vi "02 - Basic and Advanced DSP.vi"   [LabVIEW 2021]
uses:
  <vilib>/Analysis/NI_AALBase.lvlib
  <vilib>/Analysis/NI_AALPro.lvlib
  <vilib>/Analysis/NI_AAL_SigProc.lvlib
  <vilib>/gmath/NI_Gmath.lvlib
  <vilib>/addons/Digital Filter Design/NI_DigFilterLicensed.lvlib
  <vilib>/addons/_Advanced Signal Processing/NI_AdvSigProcTFA.lvlib
  <vilib>/addons/_Advanced Signal Processing/NI_AdvSigProcWA.lvlib
  <vilib>/addons/_Advanced Signal Processing/NI_AdvSigProcTSA.lvlib
  <vilib>/addons/Time Series Analysis/Correlation and Spectral Analysis.llb/TSA MUSIC (Waveform).vi
  <vilib>/Analysis/2dsp.llb/1D Convolution (DBL).vi
  <vilib>/Analysis/4window.llb/Hanning Window (DBL).vi
  <vilib>/Analysis/2dsp.llb/1D Cross Correlation (DBL).vi
  <vilib>/Analysis/3filter.llb/Chebyshev Filter (DBL).vi
  <vilib>/Analysis/2dsp.llb/Power Spectrum (DBL).vi
  <vilib>/Analysis/4window.llb/Blackman-Harris Window (DBL).vi
  <vilib>/addons/Wavelet Analysis/continuous wavelet transform.llb/WA Continuous Wavelet Transform (Waveform).vi
  <vilib>/addons/Time Frequency Analysis/Spectrogram.llb/TFA Online STFT Spectrogram (Waveform).vi
  <vilib>/addons/Time Frequency Analysis/Spectrogram.llb/TFA Choi-Williams Distribution (Waveform).vi
  <vilib>/addons/Time Series Analysis/Correlation and Spectral Analysis.llb/TSA Bispectrum (Waveform).vi
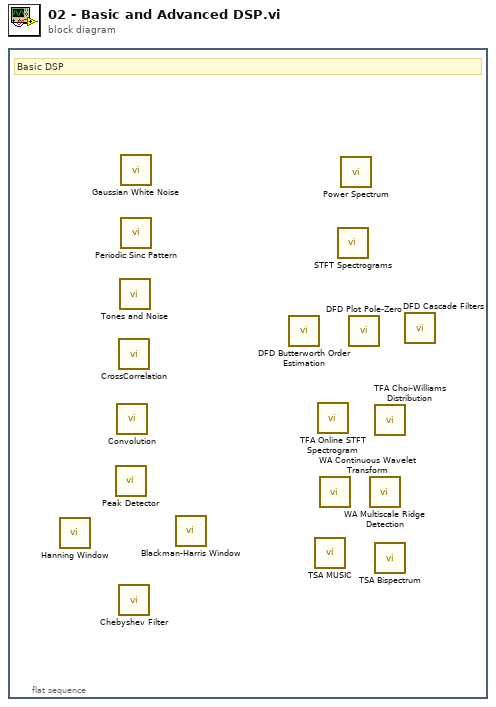
[diagram p0: block diagram]
diagram:
  n1 = flat-sequence {
    frame #0 {
      # "Basic DSP"
      n2 = call-poly <vilib>:"Hanning Window.vi"() -> ()  [unwired: 1 in, 2 out]
      n3 = call <vilib>:"Peak Detector.vi"() -> ()  [unwired: 7 in, 5 out]
      n4 = call-poly <vilib>:"Convolution.vi"() -> ()  [unwired: 10 in, 2 out]
      n5 = call-poly <vilib>:"CrossCorrelation.vi"() -> ()  [unwired: 10 in, 2 out]
      n6 = call-poly <vilib>:"Chebyshev Filter.vi"() -> ()  [unwired: 10 in, 2 out]
      n7 = call <vilib>:"Tones and Noise.vi"() -> ()  [unwired: 10 in, 2 out]
      n8 = call <vilib>:"Gaussian White Noise.vi"() -> ()  [unwired: 10 in, 2 out]
      n9 = call <vilib>:"Periodic Sinc Pattern.vi"() -> ()  [unwired: 10 in, 2 out]
      n10 = call-poly <vilib>:"Blackman-Harris Window.vi"() -> ()  [unwired: 1 in, 2 out]
      n11 = call <vilib>:"DFD Butterworth Order Estimation.vi"() -> ()  [unwired: 8 in, 4 out]
      n12 = call-poly <vilib>:"TSA MUSIC.vi"() -> ()  [unwired: 9 in, 3 out]
      n13 = call-poly <vilib>:"TFA Online STFT Spectrogram.vi"() -> ()  [unwired: 9 in, 3 out]
      n14 = call-poly <vilib>:"WA Continuous Wavelet Transform.vi"() -> ()  [unwired: 9 in, 3 out]
      n15 = call <vilib>:"STFT Spectrograms.vi"() -> ()  [unwired: 10 in, 2 out]
      n16 = call-poly <vilib>:"Power Spectrum.vi"() -> ()  [unwired: 1 in, 2 out]
      n17 = call <vilib>:"DFD Plot Pole-Zero.vi"() -> ()  [unwired: 9 in, 3 out]
      n18 = call <vilib>:"WA Multiscale Ridge Detection.vi"() -> ()  [unwired: 10 in, 2 out]
      n19 = call-poly <vilib>:"TFA Choi-Williams Distribution.vi"() -> ()  [unwired: 9 in, 3 out]
      n20 = call-poly <vilib>:"TSA Bispectrum.vi"() -> ()  [unwired: 11 in, 5 out]
      n21 = call <vilib>:"DFD Cascade Filters.vi"() -> ()  [unwired: 10 in, 2 out]
    }
  }
